vi "Refresh Item.vi"(8 "error in (no error)":errorcluster, 10 "TreeItem Index":i32, 11 "BetterTreeHandle in":refnum<class "BetterTreeHandle.lvclass">) -> (0 "error out":errorcluster, 3 "BetterTreeHandle out":refnum<class "BetterTreeHandle.lvclass">)   [LabVIEW 2020, in "BetterDragAndDrop.lvlib" / "BetterTreeHandle.lvclass"]
uses:
  BetterTreeHandle.lvclass
  C:/Code/GITHUB/BetterDragAndDrop/Source/Classes/BetterHandle/BetterHandle.lvclass
  BetterHandle/BetterHandle.lvclass/BetterHandle.ctl
  BetterTreeHandle.lvclass/BetterTreeHandle.ctl
  BetterHandle/BetterHandle.lvclass
  BetterTreeItem/BetterItem.lvclass
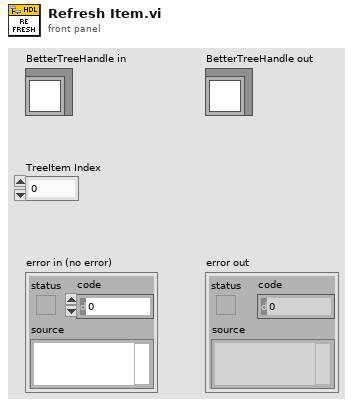
[diagram p1: front panel]
types:
  T1 = typedef "BetterDragAndDrop.lvlib/BetterTreeHandle.lvclass/TreeItem.ctl" = cluster{"Left Cell String":string, "Child Text":string[], "Child Tag":string, "Item Indent":i32, "Child Only?":bool, "Glyph Index":i32, "Font Color":u32}
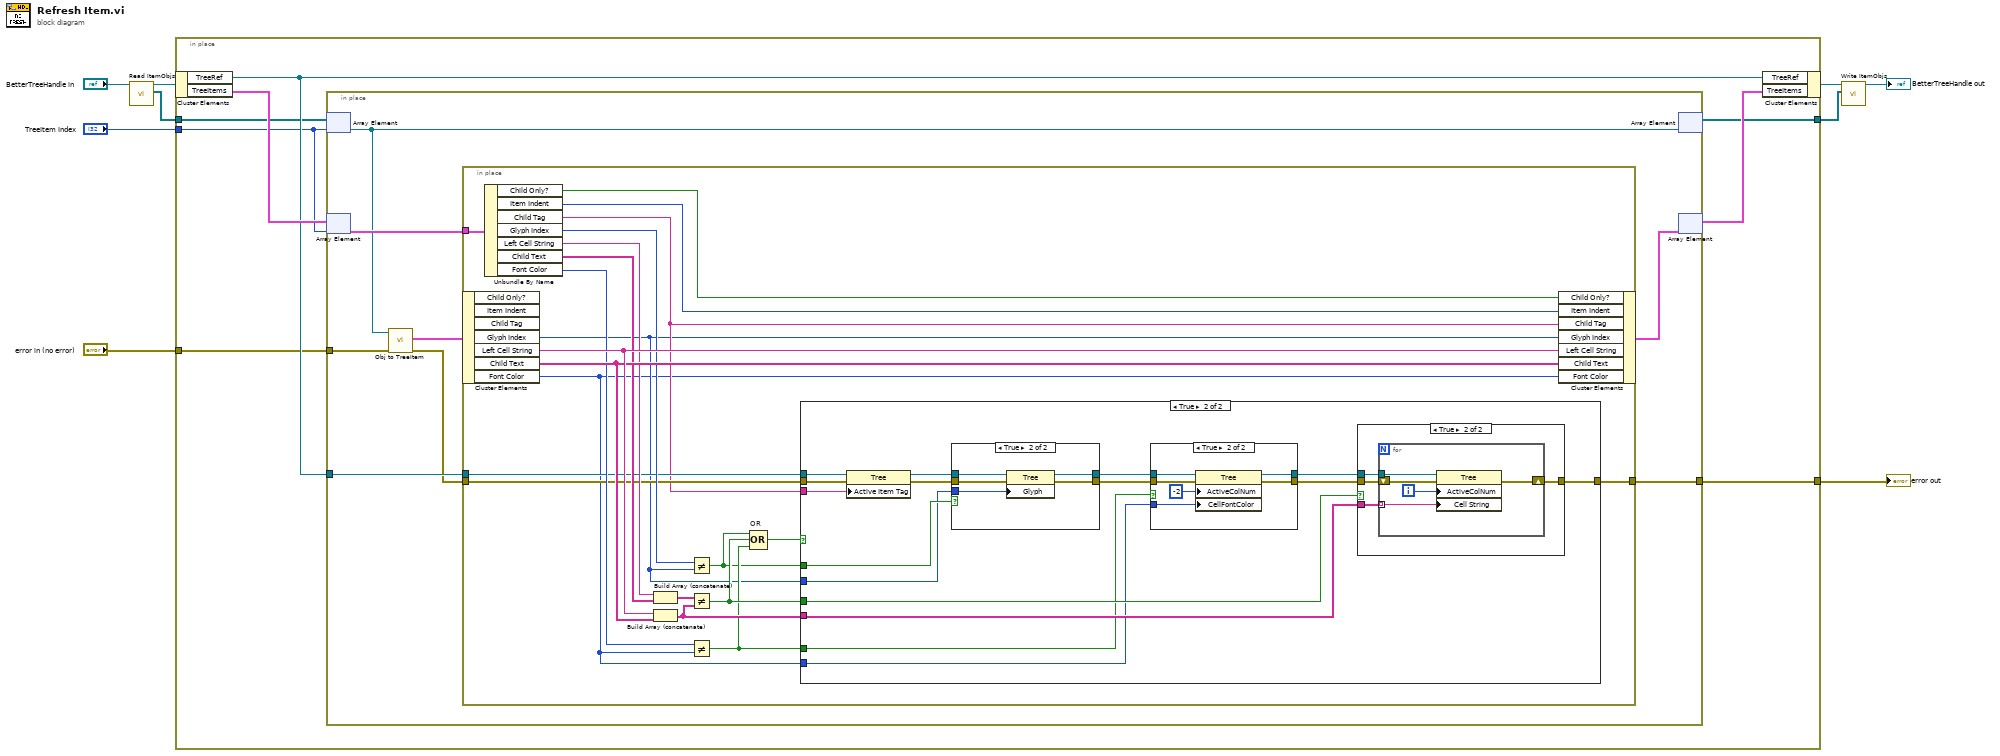
[diagram p0: block diagram]
diagram:
  n1 = call "Read ItemObjs.vi"("BetterHandle in"="BetterTreeHandle in") -> ("ItemObjs"=w4:refnum<class "BetterItem.lvclass">[], "BetterHandle out"=w5:refnum<class "BetterTreeHandle.lvclass">)  [unwired: 9 in]
  n2 = in-place {
    in-place-border: "error in (no error)" -> [w14]
    in-place-border: [w13] -> w7
    in-place-border: "TreeItem Index" -> [w12]
    in-place-border: w4 -> [w11]
    in-place-border: [w10] -> w1
    n3 = in-place-cluster #1(w5) -> ("TreeRef"=w15:refnum<vi>, "TreeItems"=w17:T1[])
    n4 = in-place {
      in-place-border: w15 -> [w25]
      in-place-border: w14 -> [w19]
      in-place-border: [w24] -> w13
      n5 = in-place-array #2(w11, w12) -> (w21:refnum<class "BetterItem.lvclass">)
      n6 = in-place-array #3(w17, w12) -> (w23:T1)
      n7 = call "Obj to TreeItem.vi"("error in (no error)"=w19, "BetterTreeItem in"=w21) -> ("error out"=w18:errorcluster, "Tree Control Item"=w20:T1)  [unwired: 7 in, 1 out]
      n8 = in-place {
        in-place-border: w25 -> [w33]
        in-place-border: w18 -> [w32]
        in-place-border: [w38] -> w24
        in-place-border: w23 -> [w46]
        n9 = in-place-cluster #4(w20) -> ("Glyph Index"=w27:i32, "Left Cell String"=w45:string, "Child Text"=w44:string[], "Font Color"=w26:u32)  [unwired: 3 out]
        n10 = Unbundle By Name(w46) -> ("Child Only?"=w43:bool, "Item Indent"=w42:i32, "Child Tag"=w31:string, "Glyph Index"=w35:i32, "Left Cell String"=w40:string, "Child Text"=w41:string[], "Font Color"=w36:u32)
        n11 = Build Array (concatenate)(w40, w41) -> (w39:string[])
        n12 = Build Array (concatenate)(w45, w44) -> (w37:string[])
        n13 = Not Equal?(x=w35, y=w27) -> (x != y?=w28:bool)
        n14 = Not Equal?(x=w39, y=w37) -> (x != y?=w34:bool)
        n15 = Not Equal?(x=w36, y=w26) -> (x != y?=w29:bool)
        n16 = Compound Arithmetic op=OR "OR"(w28, w34, w29) -> (w30:bool)
        n17 = case shown="True" w30 {
          tunnel: [w47 w63] -> w38
          tunnel: w37 -> [_ w62]
          tunnel: w34 -> [_ w61]
          tunnel: w33 -> [_ w60]
          tunnel: w32 -> [w47 w59]
          tunnel: w31 -> [_ w58]
          tunnel: w29 -> [_ w57]
          tunnel: w26 -> [_ w56]
          tunnel: w28 -> [_ w51]
          tunnel: w27 -> [_ w50]
          frame False {
          }
          frame True {
            n18 = property class="Tree"(reference=w60, error in=w59, "Active Item Tag"=w58) -> (reference out=w53:refnum<vi>, error out=w52:errorcluster)
            n19 = case shown="True" w51 {
              tunnel: [w65 w70] -> w49
              tunnel: [w64 w69] -> w48
              tunnel: w53 -> [w65 w68]
              tunnel: w52 -> [w64 w67]
              tunnel: w50 -> [_ w66]
              frame False {
              }
              frame True {
                n20 = property class="Tree"(reference=w68, error in=w67, "Glyph"=w66) -> (reference out=w70:refnum<vi>, error out=w69:errorcluster)
              }
            }
            n21 = case shown="True" w57 {
              tunnel: [w72 w78] -> w55
              tunnel: [w71 w77] -> w54
              tunnel: w56 -> [_ w75]
              tunnel: w49 -> [w72 w74]
              tunnel: w48 -> [w71 w73]
              frame False {
              }
              frame True {
                n22 = property class="Tree"(reference=w74, error in=w73, "ActiveColNum"=-2 ("Active Cell:Active Column Number"), "CellFontColor"=w75) -> (reference out=w78:refnum<vi>, error out=w77:errorcluster)
              }
            }
            n23 = case shown="True" w61 {
              tunnel: [w79 w83] -> w63
              tunnel: w62 -> [_ w82]
              tunnel: w55 -> [_ w81]
              tunnel: w54 -> [w79 w80]
              frame False {
              }
              frame True {
                n24 = for {
                  tunnel: w81 -> [w88]
                  tunnel: w82 -> [w86] mode=indexing
                  shift-right: [w84] -> w83
                  shift-left: w80 -> [w85]
                  i -> [w87]
                  n25 = property class="Tree"(reference=w88, error in=w85, "ActiveColNum"=w87, "Cell String"=w86) -> (error out=w84:errorcluster)  [unwired: 1 out]
                }
              }
            }
          }
        }
        n26 = in-place-cluster #4("Child Only?"=w43, "Item Indent"=w42, "Child Tag"=w31, "Glyph Index"=w27, "Left Cell String"=w45, "Child Text"=w44, "Font Color"=w26) -> (w22:T1)
      }
      n27 = in-place-array #2(w21) -> (w10:refnum<class "BetterItem.lvclass">[])  [unwired: 1 out]
      n28 = in-place-array #3(w22) -> (w16:T1[])  [unwired: 1 out]
    }
    n29 = in-place-cluster #1("TreeRef"=w15, "TreeItems"=w16) -> (w3:refnum<class "BetterTreeHandle.lvclass">)
  }
  "error out" <- w7
  n30 = call "Write ItemObjs.vi"("ItemObjs"=w1, "BetterHandle in"=w3) -> ("BetterHandle out"=→"BetterTreeHandle out":refnum<class "BetterTreeHandle.lvclass">)  [unwired: 9 in]
